vi "Calculate torque per wheel.vi"(8 "Error In":errorcluster, 9 "Right Motor Status":T1, 10 "Left Motor Status":T1, 11 "\"Pedals\" Status":T2 {"Acceleration pedal" scale=0.0..100.0 scale format="%#_6f%%"; "Break pedal" scale=0.0..100.0 scale format="%#_6f%%"}) -> (0 "Error Out":errorcluster, 1 "Target Torque Right":i16(knob) scale=1000.0..-1000.0, 2 "Target Torque Left":i16(knob) scale=-1000.0..1000.0)   [LabVIEW 2016]
uses:
  Pedals Status.ctl
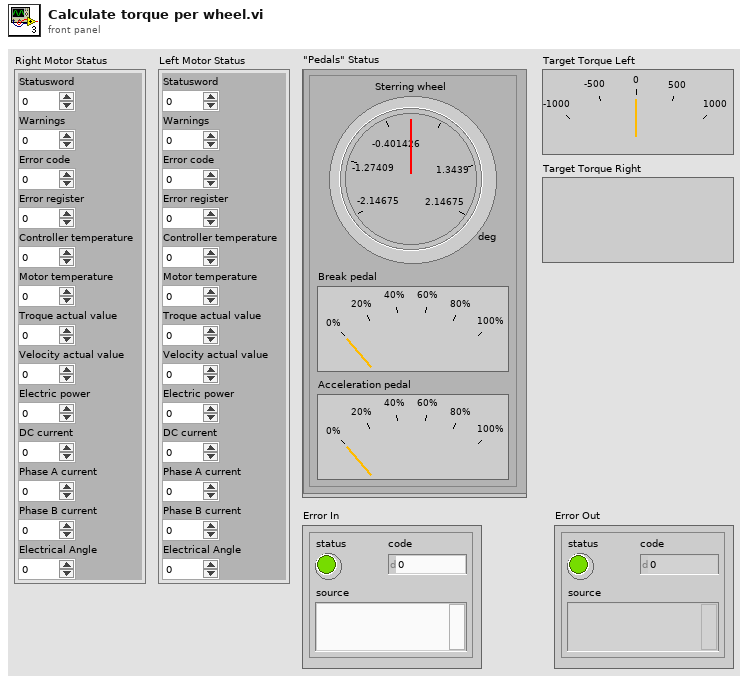
[diagram p1: front panel]
types:
  T1 = cluster{"Statusword":u16, "Warnings":u16, "Error code":u16, "Error register":u8, "Controller temperature":u8, "Motor temperature":u8, "Troque actual value":i16, "Velocity actual value":i32, "Electric power":u32, "DC current":u32, "Phase A current":u16, "Phase B current":u16, "Electrical Angle":u16}
  T2 = typedef "Pedals Status.ctl" = cluster{"Acceleration pedal":dbl, "Break pedal":dbl, "Sterring wheel":dbl[unit]}
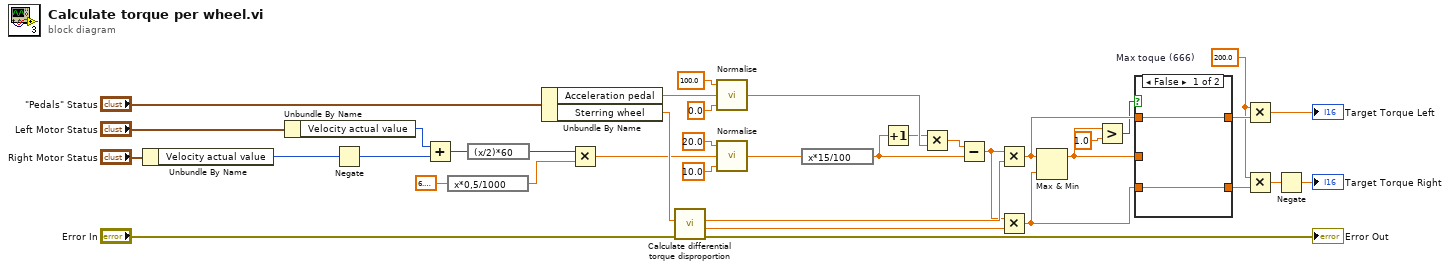
[diagram p0: block diagram]
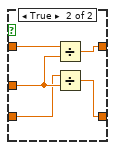
[diagram p2: hidden frame]
diagram:
  w3 = 200.0  # Max toque (666)
  n1 = Unbundle By Name("Right Motor Status") -> ("Velocity actual value"=w32:i32)
  n2 = Unbundle By Name("Left Motor Status") -> ("Velocity actual value"=w30:i32)
  n3 = Negate(x=w32) -> (-x=w31:i32)
  n4 = Add(x=w30, y=w31) -> (x+y=w28:i32)
  n5 = expression code="x*0,5/1000"(6.283185307179586) -> (w27:dbl)
  n6 = expression code="(x/2)*60"(w28) -> (w26:i32)
  n7 = Unbundle By Name("\"Pedals\" Status") -> ("Acceleration pedal"=w21:dbl, "Sterring wheel"=w25:dbl[unit])
  n8 = Multiply(x=w26, y=w27) -> (x*y=w22:dbl)
  n9 = call "Calculate differential torque disproportion.vi"("Error In"="Error In", "Steering (-123,123)"=w25) -> ("Error Out"=→"Error Out":errorcluster, "Right wheel diff scaller"=w15:dbl, "Left wheel diff scaller"=w14:dbl)  [unwired: 7 in]
  n10 = call "Normalise.vi"("min"=0.0, "value"=w21, "max"=100.0) -> ("normalised"=w16:dbl)  [unwired: 2 out]
  n11 = call "Normalise.vi"("min"=10.0 ("lower limit"), "value"=w22, "max"=20.0 ("upper limit")) -> ("normalised"=w20:dbl)  [unwired: 2 out]
  n12 = expression code="x*15/100"(w20) -> (w2:dbl)
  n13 = Increment(x=w2) -> (x+1=w1:dbl)
  n14 = Multiply(x=w1, y=w16) -> (x*y=w17:dbl)
  n15 = Subtract(x=w17, y=w2) -> (x-y=w13:dbl)
  n16 = Multiply(x=w13, y=w14) -> (x*y=w10:dbl)
  n17 = Multiply(x=w13, y=w15) -> (x*y=w9:dbl)
  n18 = Max & Min(x=w10, y=w9) -> (max(x,y)=w11:dbl)  [unwired: 1 out]
  n19 = Greater?(x=w11, y=1.0) -> (0:w8:bool)
  n20 = case shown="False" w8 {
    tunnel: w11 -> [_ w45]
    tunnel: w10 -> [w40 w44]
    tunnel: w9 -> [w39 w43]
    tunnel: [w39 w42] -> w6
    tunnel: [w40 w41] -> w7
    frame False {
    }
    frame True {
      n21 = Divide(x=w44, y=w45) -> (x/y=w41:dbl)
      n22 = Divide(x=w43, y=w45) -> (x/y=w42:dbl)
    }
  }
  n23 = Multiply(x=w3, y=w7) -> (x*y=→"Target Torque Left":dbl)
  n24 = Multiply(x=w3, y=w6) -> (x*y=w4:dbl)
  n25 = Negate(x=w4) -> (-x=→"Target Torque Right":dbl)
